vi "Format Packet Bytes.vi"(11 "frame data":u8[](array[numeric])) -> (3 "spreadsheet string":string)   [LabVIEW 2025, in "Automotive Ethernet Bus Monitor.lvclass"]
uses:
  Automotive Ethernet Bus Monitor/Automotive Ethernet Bus Monitor.lvclass
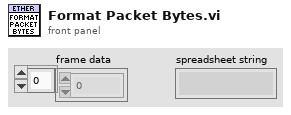
[diagram p1: front panel]
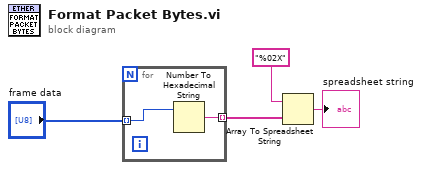
[diagram p0: block diagram]
diagram:
  n1 = for {
    tunnel: "frame data" -> [w6] mode=indexing
    tunnel: [w5] -> w4 mode=indexing
    n2 = Number To Hexadecimal String(2:w6) -> (0:w5:string)  [unwired: 1 in]
  }
  n3 = Array To Spreadsheet String(array=w4, 3:"%02X" ("format string")) -> (spreadsheet string=→"spreadsheet string":string)  [unwired: 1 in]
